vi "Shift Half Rectangle.vi"(11 "image data in":T1) -> (3 "image data out":T1)   [LabVIEW 2018]
uses:
  <vilib>/picture/picture.llb/imagedata.ctl
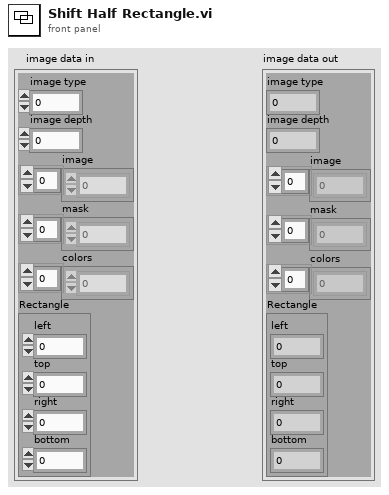
[diagram p1: front panel]
types:
  T1 = typedef "imagedata.ctl" = cluster{"image type":i32, "image depth":i32, "image":u8[], "mask":u8[], "colors":u32[], "Rectangle":cluster{"left":i16, "top":i16, "right":i16, "bottom":i16}}
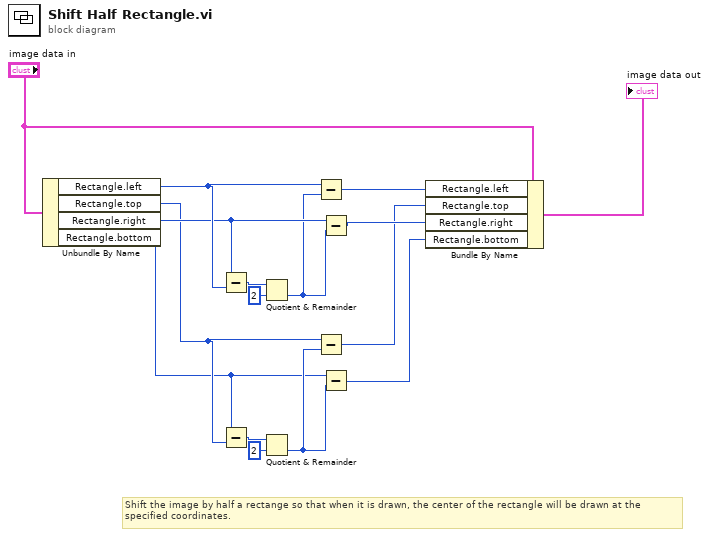
[diagram p0: block diagram]
diagram:
  # "Shift the image by half a rectange so that when it is drawn, the center of the rectangle will be drawn at the\nspecified coordinates."
  n1 = Unbundle By Name("image data in") -> ("Rectangle.left"=w13:i16, "Rectangle.top"=w5:i16, "Rectangle.right"=w11:i16, "Rectangle.bottom"=w4:i16)
  n2 = Subtract(x=w11, y=w13) -> (x-y=w15:i16)
  n3 = Subtract(x=w4, y=w5) -> (x-y=w6:i16)
  n4 = Quotient & Remainder(x=w15, y=i16 2) -> (floor(x/y)=w10:i16)  [unwired: 1 out]
  n5 = Quotient & Remainder(x=w6, y=i16 2) -> (floor(x/y)=w8:i16)  [unwired: 1 out]
  n6 = Subtract(x=w13, y=w10) -> (x-y=w12:i16)
  n7 = Subtract(x=w5, y=w8) -> (x-y=w3:i16)
  n8 = Subtract(x=w11, y=w10) -> (x-y=w9:i16)
  n9 = Subtract(x=w4, y=w8) -> (x-y=w2:i16)
  n10 = Bundle By Name(cluster="image data in", "Rectangle.left"=w12, "Rectangle.top"=w3, "Rectangle.right"=w9, "Rectangle.bottom"=w2) -> (→"image data out":T1)
